vi "mask_array.vi"(8 "error in (no error)":errorcluster, 9 "Test":u8[][](array[numeric])=[[0, 32, 0, 0, 0, 0, 0, 0], [255, 255, 255, 255, 127, 127, 127, 127], [255, 255, 255, 255, 127, 127, 127, 127], [255, 255, 255, 255, 127, 127, 127, 127]] format="%08b", 10 "下拉列表":u16(ring)=1 items=["default", "Test", "NormalUse"], 11 "address":string[](array[string])=["192.168.10.32"]) -> (0 "error out":errorcluster)   [LabVIEW 2017]
panel:
  out "Test 2":u8[](array[numeric])=[0, 32, 0, 0, 0, 0, 0, 0]
  in  "Default":u8[][](array[numeric])=[[0, 0, 0, 0], [0, 0, 0, 0]] format="%b"
  in  "Use":u8[][](array[numeric])=[[0, 0, 0, 0], [0, 0, 0, 0]] format="%b"
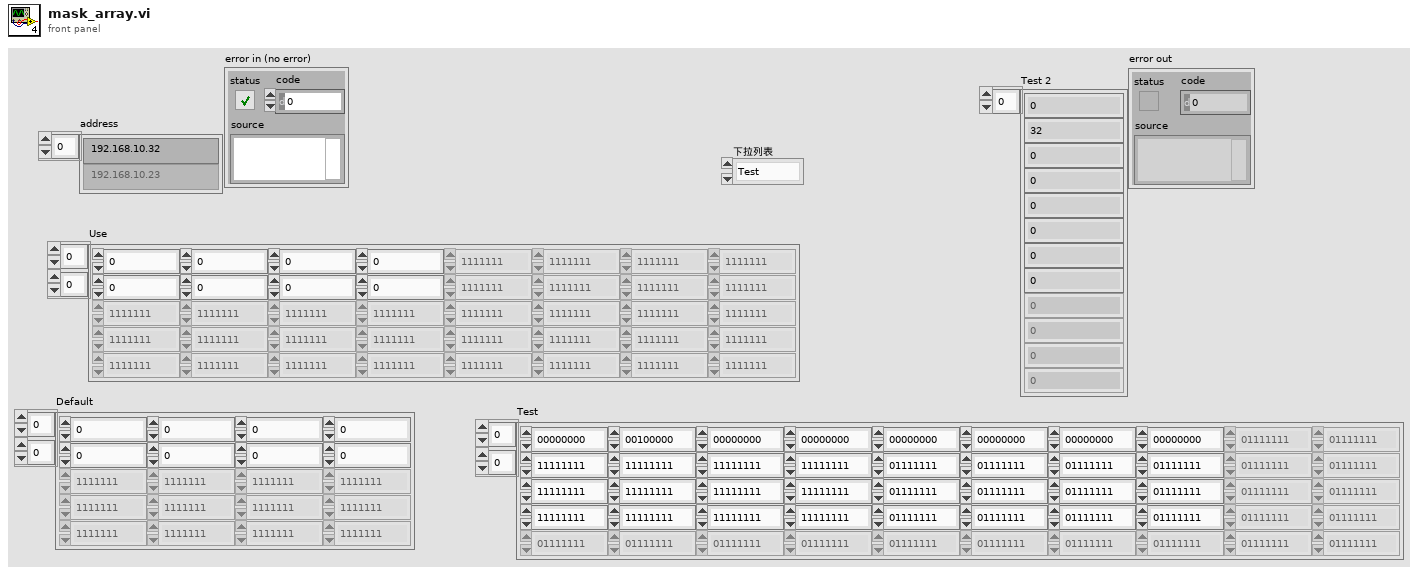
[diagram p1: front panel]
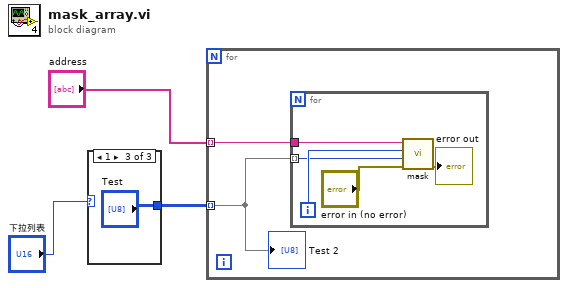
[diagram p0: block diagram]
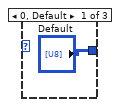
[diagram p2: hidden frame]
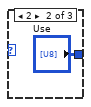
[diagram p3: hidden frame]
diagram:
  n1 = case shown="1" "下拉列表" {
    tunnel: ["Default" "Use" "Test"] -> w2
    frame 0, Default {
    }
    frame 2 {
    }
    frame 1 {
    }
  }
  n2 = for {
    tunnel: "address" -> [w8] mode=indexing
    tunnel: w2 -> [w7] mode=indexing
    n3 = for {
      tunnel: w8 -> [w13]
      tunnel: w7 -> [w11] mode=indexing
      i -> [w12]
      n4 = call "mask.vi"("error in (no error)"="error in (no error)", "mask channel"=w11, "Address"=w12, "IP address"=w13) -> ("error out"=→"error out":errorcluster)  [unwired: 7 in]
    }
    "Test 2" <- w7
  }
